vi "RichTextDemo2.vi"() -> ()   [LabVIEW 2012]
uses:
  RichTextClass/RichText.lvclass
  System.Windows.Forms
panel:
  out "Lines":string[](array[string])
  out "Rtf":string
  in  "text":string="\nCsx"
  in  "停止":bool
  in  "RichTextBox":refnum<k24>(container)
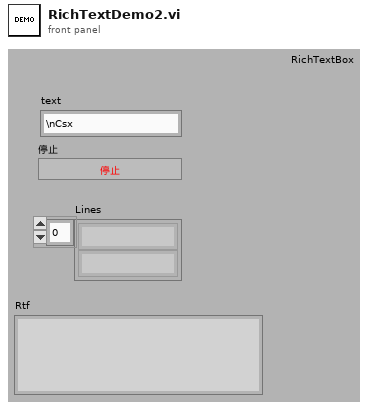
[diagram p1: front panel]
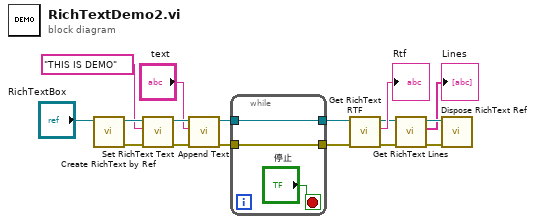
[diagram p0: block diagram]
diagram:
  n1 = call "Create RichText by Ref.vi"("RichTextBox"="RichTextBox") -> ("error out"=w15:errorcluster, "RichText 输出"=w16:refnum<class "RichText.lvclass">)  [unwired: 9 in]
  n2 = call "Set RichText Text.vi"("error in (no error)"=w15, "Text"="THIS IS DEMO", "RichText 输入"=w16) -> ("error out"=w12:errorcluster, "RichText 输出"=w13:refnum<class "RichText.lvclass">)  [unwired: 7 in]
  n3 = call "Append Text.vi"("error in (no error)"=w12, "text"="text", "RichText 输入"=w13) -> ("error out"=w9:errorcluster, "RichText 输出"=w10:refnum<class "RichText.lvclass">)  [unwired: 7 in]
  n4 = while {
    tunnel: [w19] -> w8
    tunnel: w10 -> [w19]
    tunnel: [w18] -> w7
    tunnel: w9 -> [w18]
    stop <- "停止" stop-if-true
  }
  n5 = call "Get RichText RTF.vi"("error in (no error)"=w7, "RichText 输入"=w8) -> ("error out"=w4:errorcluster, "Rtf"=→"Rtf":string, "RichText 输出"=w5:refnum<class "RichText.lvclass">)  [unwired: 7 in]
  n6 = call "Get RichText Lines.vi"("error in (no error)"=w4, "RichText 输入"=w5) -> ("error out"=w3:errorcluster, "Lines"=→"Lines":string[], "RichText 输出"=w2:refnum<class "RichText.lvclass">)  [unwired: 7 in]
  n7 = call "Dispose RichText Ref.vi"("error in (no error)"=w3, "RichText 输入"=w2) -> ()  [unwired: 8 in, 2 out]
